vi "TENMA 72-2930 output enable with settings.vi"(6 "Initial wait (ms)":u32=3000, 8 "Running current limit (A)":sgl=5.0, 9 "Initial current limit (A)":sgl=10.0, 10 "Voltate output (V)":sgl=24.0, 11 "Port":refnum<visa-resource-name>) -> (0 "Returned current limit (A)":sgl=nan format="%_4g", 1 "Returned voltage output (V)":sgl=nan format="%_4g", 2 "CV mode":bool, 3 "Output enabled":bool, 4 "Error out":errorcluster)   [LabVIEW 2017]
uses:
  ctls/TENMA 72-2xxx commands.ctl
panel:
  # "PN 23/04/18"
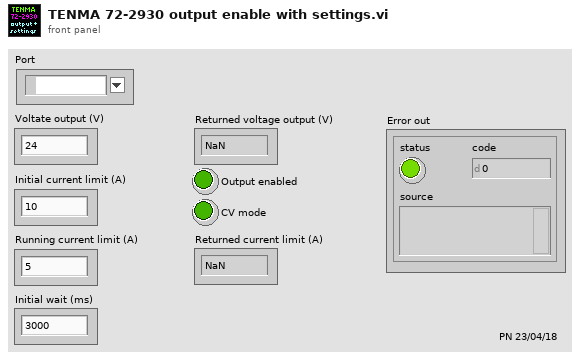
[diagram p1: front panel]
types:
  T1 = typedef "TENMA 72-2xxx commands.ctl" = string
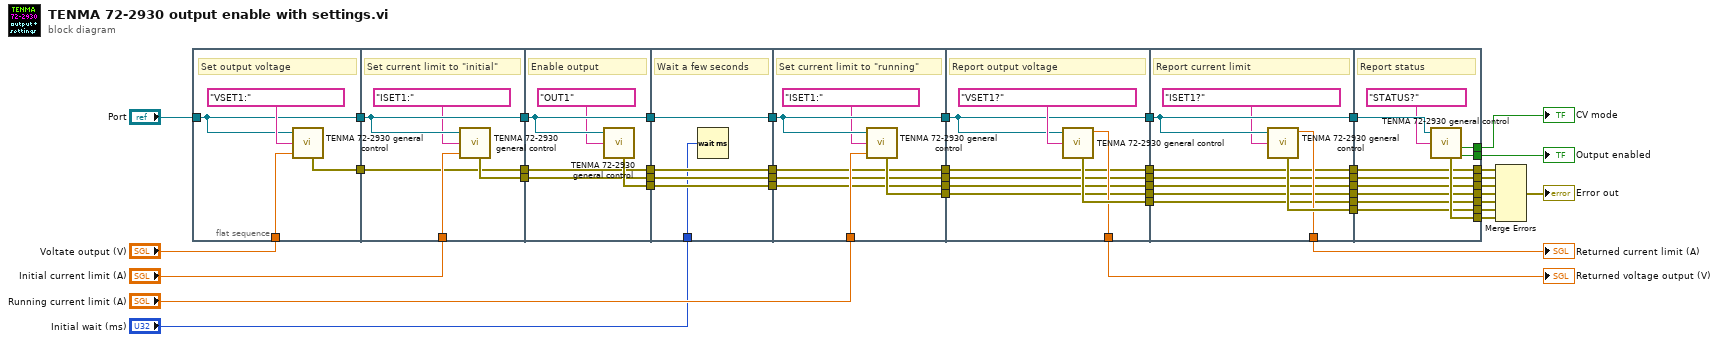
[diagram p0: block diagram]
diagram:
  n1 = flat-sequence {
    tunnel: "Port" -> [w51]
    tunnel: [w51] -> w43
    tunnel: [w50] -> w40
    tunnel: "Voltate output (V)" -> [w49]
    tunnel: [w57] -> w45
    tunnel: w43 -> [w57]
    tunnel: w40 -> [w53]
    tunnel: [w55] -> w39
    tunnel: "Initial current limit (A)" -> [w54]
    tunnel: [w53] -> w2
    tunnel: [w62] -> w46
    tunnel: w45 -> [w62]
    tunnel: w39 -> [w59]
    tunnel: [w60] -> w38
    tunnel: [w59] -> w9
    tunnel: [w58] -> w3
    tunnel: w2 -> [w58]
    tunnel: [w67] -> w47
    tunnel: w46 -> [w67]
    tunnel: w38 -> [w66]
    tunnel: [w66] -> w15
    tunnel: [w65] -> w10
    tunnel: w9 -> [w65]
    tunnel: [w64] -> w4
    tunnel: w3 -> [w64]
    tunnel: "Initial wait (ms)" -> [w63]
    tunnel: [w74] -> w42
    tunnel: w47 -> [w74]
    tunnel: [w72] -> w37
    tunnel: "Running current limit (A)" -> [w71]
    tunnel: [w70] -> w16
    tunnel: w15 -> [w70]
    tunnel: [w69] -> w11
    tunnel: w10 -> [w69]
    tunnel: [w68] -> w5
    tunnel: w4 -> [w68]
    tunnel: w42 -> [w81]
    tunnel: [w81] -> w41
    tunnel: w37 -> [w78]
    tunnel: [w80] -> w36
    tunnel: [w79] -> w31
    tunnel: [w78] -> w20
    tunnel: [w77] -> w17
    tunnel: w16 -> [w77]
    tunnel: [w76] -> w12
    tunnel: w11 -> [w76]
    tunnel: [w75] -> w6
    tunnel: w5 -> [w75]
    tunnel: w41 -> [w91]
    tunnel: [w91] -> w44
    tunnel: w36 -> [w87]
    tunnel: [w89] -> w35
    tunnel: [w88] -> w30
    tunnel: [w87] -> w23
    tunnel: [w86] -> w21
    tunnel: w20 -> [w86]
    tunnel: [w85] -> w18
    tunnel: w17 -> [w85]
    tunnel: [w84] -> w13
    tunnel: w12 -> [w84]
    tunnel: [w83] -> w7
    tunnel: w6 -> [w83]
    tunnel: w44 -> [w102]
    tunnel: w35 -> [w97]
    tunnel: [w100] -> w26
    tunnel: [w99] -> w28
    tunnel: [w98] -> w29
    tunnel: [w97] -> w25
    tunnel: [w96] -> w24
    tunnel: w23 -> [w96]
    tunnel: [w95] -> w22
    tunnel: w21 -> [w95]
    tunnel: [w94] -> w19
    tunnel: w18 -> [w94]
    tunnel: [w93] -> w14
    tunnel: w13 -> [w93]
    tunnel: [w92] -> w8
    tunnel: w7 -> [w92]
    frame #0 {
      # "Set output voltage"
      n2 = call "TENMA 72-2930 general control.vi"("Value to set"=w49, "Command"=T1 "VSET1:", "Port"=w51) -> ("error out"=w50:errorcluster)  [unwired: 1 in, 4 out]
    }
    frame #1 {
      # "Set current limit to \"initial\""
      n3 = call "TENMA 72-2930 general control.vi"("Value to set"=w54, "Command"=T1 "ISET1:", "Port"=w57) -> ("error out"=w55:errorcluster)  [unwired: 1 in, 4 out]
    }
    frame #2 {
      # "Enable output"
      n4 = call "TENMA 72-2930 general control.vi"("Command"=T1 "OUT1", "Port"=w62) -> ("error out"=w60:errorcluster)  [unwired: 2 in, 4 out]
    }
    frame #3 {
      # "Wait a few seconds"
      n5 = Wait (ms)(milliseconds to wait=w63) -> ()  [unwired: 1 out]
    }
    frame #4 {
      # "Set current limit to \"running\""
      n6 = call "TENMA 72-2930 general control.vi"("Value to set"=w71, "Command"=T1 "ISET1:", "Port"=w74) -> ("error out"=w72:errorcluster)  [unwired: 1 in, 4 out]
    }
    frame #5 {
      # "Report output voltage"
      n7 = call "TENMA 72-2930 general control.vi"("Command"=T1 "VSET1?", "Port"=w81) -> ("error out"=w80:errorcluster, "Returned value"=w79:sgl)  [unwired: 2 in, 3 out]
    }
    frame #6 {
      # "Report current limit"
      n8 = call "TENMA 72-2930 general control.vi"("Command"=T1 "ISET1?", "Port"=w91) -> ("error out"=w89:errorcluster, "Returned value"=w88:sgl)  [unwired: 2 in, 3 out]
    }
    frame #7 {
      # "Report status"
      n9 = call "TENMA 72-2930 general control.vi"("Command"=T1 "STATUS?", "Port"=w102) -> ("Output enabled"=w98:bool, "error out"=w100:errorcluster, "CV mode"=w99:bool)  [unwired: 2 in, 2 out]
    }
  }
  n10 = Merge Errors(w8, w14, w19, w22, w24, w25, w26) -> (→"Error out":errorcluster)
  "Returned voltage output (V)" <- w31
  "Returned current limit (A)" <- w30
  "Output enabled" <- w29
  "CV mode" <- w28
